vi "SPA.vi"(0 "System no.":i32=1 min=1 max=4 step=1, 2 "Axis to set":string[](array[string]), 3 "Parameter value":dbl[](array[numeric]) format="%.6f", 4 "No.of digits":i16=4, 5 "error in":errorcluster, 6 "Parameter number":i32[](array[numeric]), 7 "Parameter no. format \n(Decimal: FALSE)":bool, 8 "Parameter number (hex)":u32[](array[numeric]) format="%.0x", 9 "Parameter format \n(Num.: FALSE)":bool, 10 "Parameter string":string[](array[string])) -> (14 "Controller error":bool, 19 "error out":errorcluster)   [LabVIEW 2020]
doc: "Sets parameters, waits 100 ms and queries ERR?. For axis-related parameters, Axis to set is the axis name, for piezo-, sensor, PIShift or demux-related parameters, the channel number, otherwise a parameter-related code. If parameter no. is in decimal format, use \"Parameter number\" input, for hexadecimal parameter numbers use \"Parameter number (hex)\" input and switch \"Parameter no. format\" to TRUE. For numeric parameter values use \"Parameter value\" input, for parameter strings use \"Parameter string\" input and switch \"Parameter format\" to TRUE. Do not mix decimal and hex. parameter numbers or numeric and string parameter values in one call. Parameter numbers which can be set depend on current CCL level. See GCS DLL manual for available parameter numbers and values. No. of digits is the number of digits after the decimal point in the numeric parameter value(s) that will be sent. Controller error is TRUE if selected system reports an error code which is not 0. \n\nC-413, C-867, C-877, C-884, C-886, E-135, E-516, E-517, E-518, C-891, E-710, E-712, E-725, E-727, E-753, E-754, E-755, E-861, E-870, E-871, E-872, E-873, E-874, Hydra, Pollux, Mercury_GCS: The SPAcommand saves the parameters in RAM only. To save the currently valid parameters to flash ROM, where they become the power-on defaults, you must run WPA.vi. Parameter changes not saved with WPA will be lost when the controller is powered off.\n\nC-413: Parameter no. format is TRUE (hex.). Use HPA?.vi to get valid parameter numbers or see the C-413 user manual. Do not set more than 4 parameters at once. \n\nC-702: Parameter no. format is FALSE (decimal). \nWARNING: This command is for setting hardware-specific parameters. Wrong values may lead to improper operation or damage of your hardware! Change settings only after consultation with PI.\n\nC-843: Parameter no. format is FALSE (decimal). WARNING \nThis command is primarily for setting hardware-specific parameters of non-PI stages connected to the controller. Please refer to the stage manual for valid parameter settings. If you have a PI stage connected, please do not change any parameters except P (1), I (2), D (3), I-limit (4) and VFF (5).\nFor precision and convenience with gearbox systems, the counts per physical unit factor can be entered as numerator and denominator of a fraction (parameters 14 and 15). \n\nC-843.PM: Parameter no. format is FALSE (decimal). See C-843 for warnings. \n\nC-865: Parameter no. format is FALSE (decimal). See C-843 for warnings. \n\nC-866: Parameter no. format is FALSE (decimal). See C-843 for warnings. \n\nC-867, C-877: Parameter no. format is TRUE (hex.). Use HPA?.vi to get valid parameter numbers or see the controller user manual. Only one parameter value for only one axis per command allowed. \n\nC-880: Parameter no. format is FALSE (decimal). The most important parameter numbers are:\n- 1: P-term (0 to 32767)\n- 2: I-term (0 to 32767)\n- 3: D-term (0 to 32767)\n- 4: I-Limit (integration limit) (0 to 32767)\n- 5: VFF (velocity feed forward) (0 to 32767)\n- 10: maximum velocity (0 to 1.79769313486231E308)\n- 11: maximum allowed acceleration (0 to 1.79769313486231E308)\n- 13: maximum allowed Jerk (- 1.79E308 to 1.79E308)\n\nC-880K005: VI only supported when called through PI_Multix.vi. See C-880 for a description of parameter numbers.\n\nC-884: Parameter no. format is TRUE (hex.). Use HPA?.vi to get valid parameter numbers or see the C-884 user manual. Do not set more than 4 parameters at once. \n\nC-891: Parameter no. format is TRUE (hex.). Use HPA?.vi to get valid parameter numbers or see the controller user manual. Do not set more than 1 parameter at once. \n\nE-516: Parameter no. format is FALSE (decimal). The following parameter numbers are valid:\n- 7: Ksen (Coefficient of Sensor K_s). When sensor output change is 1V, the position change of stage is K_s (µm). (- 3.402823466e+38F to 3.402823466e+38F)\n- 8: Osen (Offset of Sensor Os). When sensor output is 0V, the actual position of stage is Os (µm). (- 3.402823466e+38F to 3.402823466e+38F)\n- 9: Kpzt (Coefficient of PZT voltage amplifier Kpzt). When DAC output change is 1V, the PZT Voltage change is Kpzt (V) (- 3.402823466e+38F to 3.402823466e+38F)\n- 10: Opzt (Offset of PZT voltage amplifier Opzt ) When DAC output is 0V, the PZT Voltage is Opzt (V) (- 3.402823466e+38F to 3.402823466e+38F)\n- 117442816: Tolerance for ONT software emulation (µm) (0 < value < 1000)\n\nE-135: Parameter no. format is TRUE (hex.). Use HPA?.vi to get valid parameter numbers or see the controller user manual. \n\nE-517, E-518: Parameter no. format is TRUE (hex.). Use HPA?.vi to get valid parameter numbers or see the controller user manual. \n\nE-709: Parameter no. format is TRUE (hex.). Only one parameter value for only one axis per command allowed. Use HPA?.vi to get valid parameter numbers or see the E-709 user manual. \n\nE-710: Parameter no. format is TRUE (hex.). Use HPA?.vi to get valid parameter numbers or see the E7XX_GCS_DLL Manual. \n\nE-712: Parameter no. format is TRUE (hex.). Use HPA?.vi to get valid parameter numbers or see the E-712 user manual. Do not set more than 10 parameters at once. \n\nE-725: Parameter no. format is TRUE (hex.). Use HPA?.vi to get valid parameter numbers or see the E-725 user manual. Do not set more than 10 parameters at once. \n\nE-753: Parameter no. format is TRUE (hex.). Use HPA?.vi to get valid parameter numbers or see the E-753 user manual. \n\nE-754: Parameter no. format is TRUE (hex.). Use HPA?.vi to get valid parameter numbers or see the E-753 user manual. \n\nE-755: Parameter no. format is TRUE (hex.). Use HPA?.vi to get valid parameter numbers or see the E-755 user manual. \n\nE-761: Parameter no. format is TRUE (hex.). Use HPA?.vi to get valid parameter numbers or see the user manual. See E-710 for warnings. Do not set more than 10 parameters at once. \nThe SPA command saves the parameters in RAM only. To save the currently valid parameters to flash ROM, where they become the power-on defaults, you must run WPA.vi. Parameter changes not saved with WPA will be lost when the PC is powered off or the E-761 is rebooted.\n\nE-816: Parameter no. format is FALSE (decimal). See E-516 for a description of parameter numbers. This command cannot be issued to a slave. Each command limited to setting one parameter for only one axis.\n\nE-861: Parameter no. format is TRUE (hex.). Use HPA?.vi to get valid parameter numbers or see the E-861 user manual. Only one parameter value for only one axis per command allowed. The SPA command saves the parameters in RAM only. To save the currently valid parameters to flash ROM, where they become the power-on defaults, you must run WPA.vi. Parameter changes not saved with WPA will be lost when the controller is powered off.\n\nE-870: Parameter no. format is TRUE (hex.). Use HPA?.vi to get valid parameter numbers or see the E-870 user manual. Each command is limited to set one parameter for only one channel.\n\nE-871, E-872, E-873, E-874: Parameter no. format is TRUE (hex.). Use HPA?.vi to get valid parameter numbers or see the controller user manual. Only one parameter value for only one axis per command allowed. \n\nC-887, F-206, M-8X0: Parameter no. format is TRUE (hex.). Use HPA?.vi to get valid parameter numbers or see the controller user manual. Only for GCS syntax version = GCS 2.0 or higher (check with CSV?.vi. If CSV?.vi is not supported, syntax version is GCS 1.0).\n\nHydra, Pollux: Parameter no. format is TRUE (hex.). Use HPA?.vi to get valid parameter numbers or see the GCS DLL user manual. Do not set more than 10 parameters at once. \n\nMercury: Parameter no. format is FALSE (decimal). See C-843 for warnings. The SPA command saves the parameters in RAM only. Use PIStageEditor to change parameters or add new stages to the data base permanently.\n\nMercury_GCS: Parameter no. format is TRUE (hex.). Use HPA?.vi to get valid parameter numbers or see the Mercury user manual. Only one parameter value for only one axis per command allowed. \n\nWarning: This command is for setting hardware-specific parameters. Wrong values may lead to improper operation or damage of your hardware!"
panel:
  # "This vi sets parameters, waits 100 ms and queries ERR?. If parameter no. is in decimal format, use \"Parameter no.\" input, for \nhexadecimal parameter numbers use \"Parameter no. (hex)\" input and switch \"Parameter no. format\" to TRUE. For numeric \nparameter values use \"Parameter value\" input, for parameter strings use \"Parameter string\" input and switch \"Parameter \nformat\" to TRUE. Do not mix decimal and hex. parameter numbers or numeric and string parameter values in one call. See GCS\nDLL manual for available parameter numbers and values."
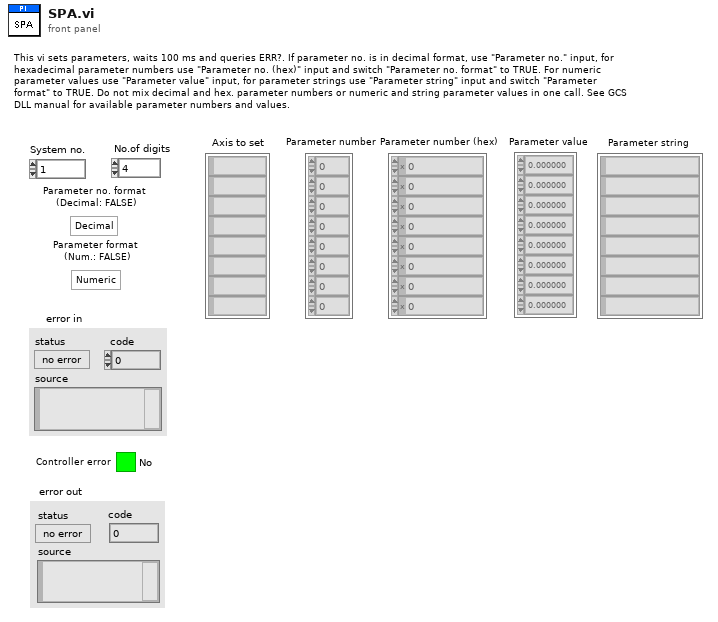
[diagram p1: front panel]
types:
  T1 = enum16{"Disable error check", "Force error check", "Use global settings"}
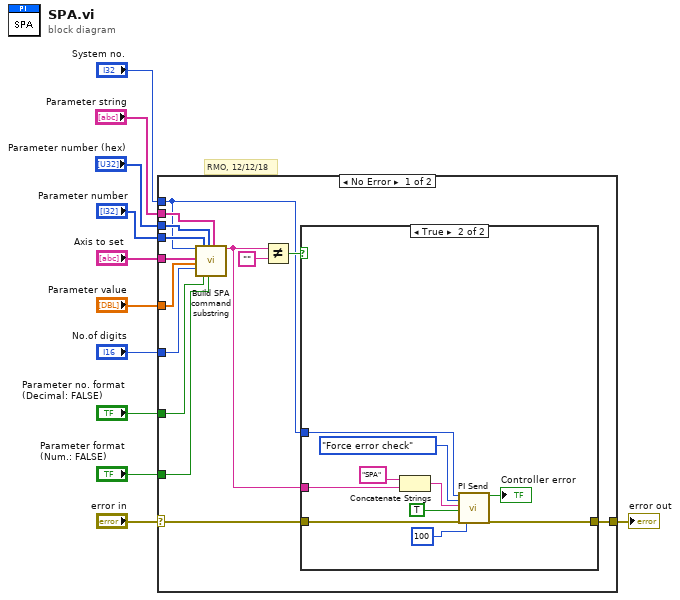
[diagram p0: block diagram]
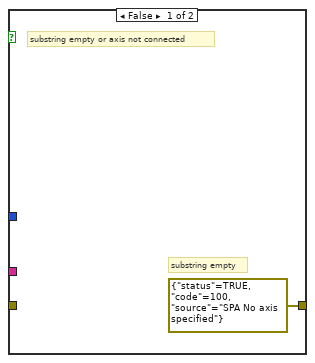
[diagram p2: hidden frame]
diagram:
  # "RMO, 12/12/18"
  n1 = case shown="No Error" "error in" {
    selector: "error in" -> [w12 w37]
    tunnel: [w25 w37] -> w11
    tunnel: "Parameter value" -> [w22 _]
    tunnel: "No.of digits" -> [w21 _]
    tunnel: "System no." -> [w15 _]
    tunnel: "Axis to set" -> [w20 _]
    tunnel: "Parameter number" -> [w19 _]
    tunnel: "Parameter string" -> [w18 _]
    tunnel: "Parameter number (hex)" -> [w17 _]
    tunnel: "Parameter no. format \n(Decimal: FALSE)" -> [w14 _]
    tunnel: "Parameter format \n(Num.: FALSE)" -> [w13 _]
    frame No Error {
      n2 = call "Build SPA command substring.vi"("System no."=w15, "Axes to set"=w20, "Parameter values"=w22, "No. of digits"=w21, "Parameter number"=w19, "Parameter no. format \n(Decimal: FALSE)"=w14, "Parameter number (hex)"=w17, "Parameter format \n(Num.: FALSE)"=w13, "Parameter strings"=w18) -> ("SPA command substring"=w23:string)  [unwired: 1 in, 9 out]
      n3 = Not Equal?(x=w23, y="") -> (x != y?=w16:bool)
      n4 = case shown="True" w16 {
        tunnel: w23 -> [_ w35]
        tunnel: [errorcluster {"status"=TRUE, "code"=100, "source"="SPA No axis specified"} ("error out") w27] -> w25
        tunnel: w12 -> [_ w32]
        tunnel: w15 -> [_ w31]
        frame False {
          # "substring empty"
          # "substring empty or axis not connected"
        }
        frame True {
          n5 = Concatenate Strings("SPA", w35) -> (w33:string)
          n6 = call "PI Send.vi"("System no."=w31, "Error check settings"=T1."Force error check", "String to send"=w33, "Attach termination char.?"=TRUE ("Attach Linefeed?"), "error in"=w32, "Delay before error check (ms)"=u32 100 ("milliseconds to wait")) -> ("Controller error"=→"Controller error":bool, "error out"=w27:errorcluster)  [unwired: 12 out]
        }
      }
    }
    frame Error {
    }
  }
  "error out" <- w11
